vi "global_process_names.vi"() -> ()   [LabVIEW 2011, in "Fiberscope_library.lvlib"]
uses:
  Fiberscope_library.lvlib
panel:
  in  "Process_names":string[](array[string])=["DAQ", "pixel_mapper", "averager", "display", "pockels", "storage"]
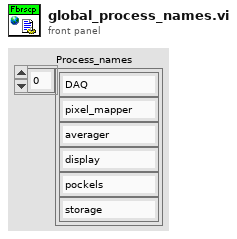
[diagram p1: front panel]
diagram:
